vi "Copy Image To Pixmap.vi"(8 "error in (no error)":errorcluster, 11 "image_ptr":i64) -> (0 "error out":errorcluster, 3 "Image":T1)   [LabVIEW 2020, in "G-Image.lvlib"]
doc: "Read the image data from the pointer into LabVIEW, then free the mmeory. The image is returned as a LabVIEW pixmap."
uses:
  G-Image.lvlib
  <vilib>/picture/picture.llb/imagedata.ctl
  <vilib>/Utility/error.llb/Error Cluster From Error Code.vi
  lib/g_image_32.dll
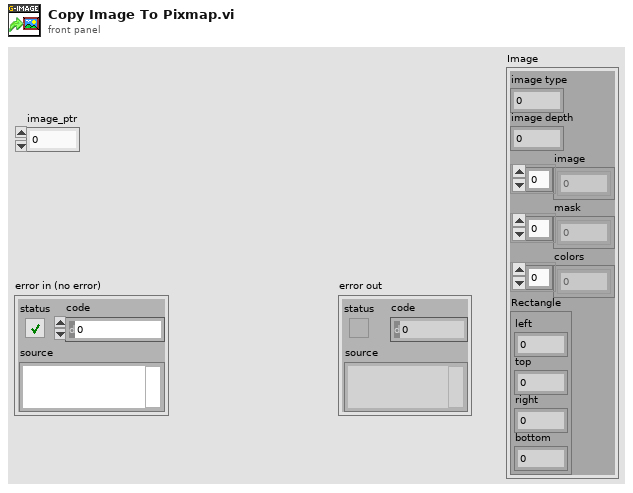
[diagram p1: front panel]
types:
  T1 = typedef "imagedata.ctl" = cluster{"image type":i32, "image depth":i32, "image":u8[], "mask":u8[], "colors":u32[], "Rectangle":cluster{"left":i16, "top":i16, "right":i16, "bottom":i16}}
  T2 = cluster{"data":i32, "data_size":u32, "width":u32, "height":u32, "depth":u32}
  T3 = cluster{"data":i64, "data_size":u32, "width":u32, "height":u32, "depth":u32}
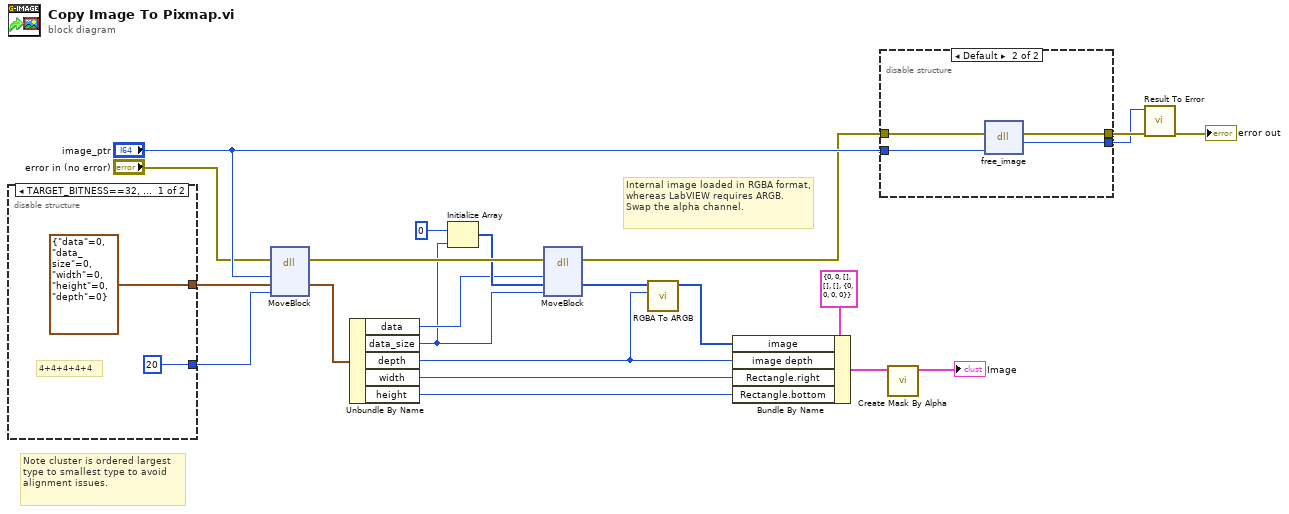
[diagram p0: block diagram]
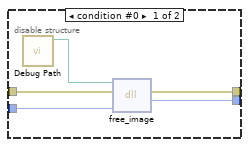
[diagram p2: hidden frame]
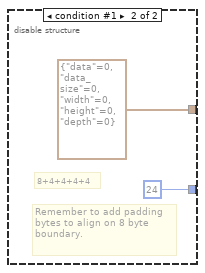
[diagram p3: hidden frame]
diagram:
  # "Internal image loaded in RGBA format, whereas LabVIEW requires ARGB. Swap the alpha channel."
  # "Note cluster is ordered largest type to smallest type to avoid alignment issues."
  n1 = disable-structure shown="TARGET_BITNESS==32, Default" {
    disable-tunnel: [T2 {"data"=0, "data_size"=0, "width"=0, "height"=0, "depth"=0} T3 {"data"=0, "data_size"=0, "width"=0, "height"=0, "depth"=0}] -> w14
    disable-tunnel: [20 ("x") 24 ("x")] -> w17
    frame condition #0 (active) {
      # "4+4+4+4+4"
    }
    frame condition #1 {
      # "Remember to add padding bytes to align on 8 byte boundary."
      # "8+4+4+4+4"
    }
  }
  n2 = dll-call lib="LabVIEW" fn="MoveBlock"(error in="error in (no error)", "Address (Pointer)"="image_ptr", "Destination"=w14, "Size"=w17) -> (error out=w18:errorcluster, "Destination"=w16:T2)  [unwired: 5 in, 1 out]
  n3 = Unbundle By Name(w16) -> ("data"=w11:i32, "data_size"=w8:u32, "depth"=w3:u32, "width"=w10:u32, "height"=w9:u32)
  n4 = Initialize Array(u8 0 ("element"), w8) -> (w12:u8[])
  n5 = dll-call lib="LabVIEW" fn="MoveBlock"(error in=w18, "Address (Pointer)"=w11, "Destination"=w12, "Size"=w8) -> (error out=w15:errorcluster, "Destination"=w4:u8[])  [unwired: 5 in, 1 out]
  n6 = call "RGBA To ARGB.vi"("Depth"=w3, "RGBA"=w4) -> ("ARGB"=w2:u8[])  [unwired: 9 in]
  n7 = Bundle By Name(cluster=T1 {"image type"=0, "image depth"=0, "image"=[], "mask"=[], "colors"=[], "Rectangle"={"left"=0, "top"=0, "right"=0, "bottom"=0}} ("Pixmap"), "image"=w2, "image depth"=w3, "Rectangle.right"=w10, "Rectangle.bottom"=w9) -> (w6:T1)
  n8 = disable-structure shown="Default" {
    disable-tunnel: w15 -> [w30 w35]
    disable-tunnel: [w29 w34] -> w20
    disable-tunnel: [w28 w33] -> w19
    disable-tunnel: "image_ptr" -> [w27 w32]
    frame condition #0 {
      n9 = call "Debug Path.vi"() -> ("Debug Path"=w31:path)  [unwired: 11 in]
      n10 = dll-call lib="?" fn="free_image"(path in=w31, error in=w30, "image_ptr"=w27) -> (error out=w29:errorcluster, "result"=w28:i32)  [unwired: 2 in, 1 out]
    }
    frame condition #1 (active) {
      n11 = dll-call lib="C:/github/dataflowg/g-image/src/LabVIEW/G-Image/lib/g_image_*.*" fn="free_image"(error in=w35, "image_ptr"=w32) -> (error out=w34:errorcluster, "result"=w33:i32)  [unwired: 3 in, 1 out]
    }
  }
  n12 = call <vilib>:"Create Mask By Alpha.vi"("image data"=w6) -> ("masked image data"=→"Image":T1)  [unwired: 10 in]
  n13 = call "Result To Error.vi"("error in (no error)"=w20, "Result Code"=w19) -> ("error out"=→"error out":errorcluster)  [unwired: 9 in]
